vi "Image.vi"(2 "XRef":refnum<vi>, 3 "State In":T1={"Input Type"=variant(dbl 0.0), "Selection"=0, "Element Names"=[], "Type Strings"=[], "Element Types"=[]}) -> (0 "Image":picture)   [LabVIEW 2015, in "Construct-Tagged-Union.xnode"]
doc: "This ability VI is used to describe your XNode's appearance. The origin of Image corresponds to the top-left corner of your XNode. The bounds of your XNode are used to crop this image. If you want LabVIEW to update your image, you need to inform it through the UpdateImage or UpdateImageAndBounds replies. Any areas where you do not draw are transparent, so regions intended to appear white should be explicitly drawn.\n \n Remember to localize any strings that are part of your image.\n\nDefault behavior: None.\n\nThis ability does not provide UI and OS messages are not handled."
uses:
  Construct-Tagged-Union.xnode
  State.ctl
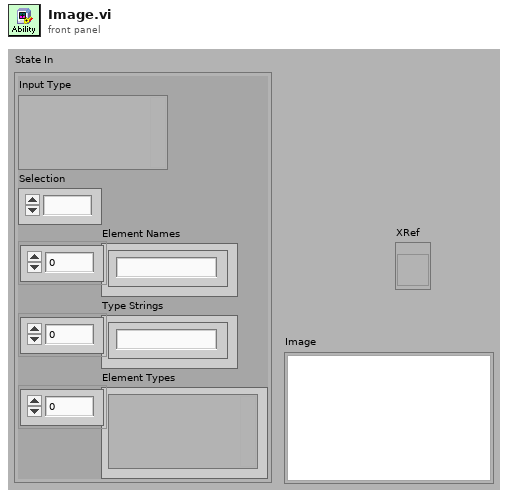
[diagram p1: front panel]
types:
  T1 = typedef "Construct-Tagged-Union.xnode/State.ctl" = cluster{"Input Type":variant, "Selection":i32, "Element Names":string[], "Type Strings":string[], "Element Types":variant[]}
  T2 = typedef "imagedata.ctl" = cluster{"image type":i32, "image depth":i32, "image":u8[], "mask":u8[], "colors":u32[], "Rectangle":cluster{"left":i16, "top":i16, "right":i16, "bottom":i16}}
  T3 = cluster{"left":i16, "top":i16, "right":i16, "bottom":i16}
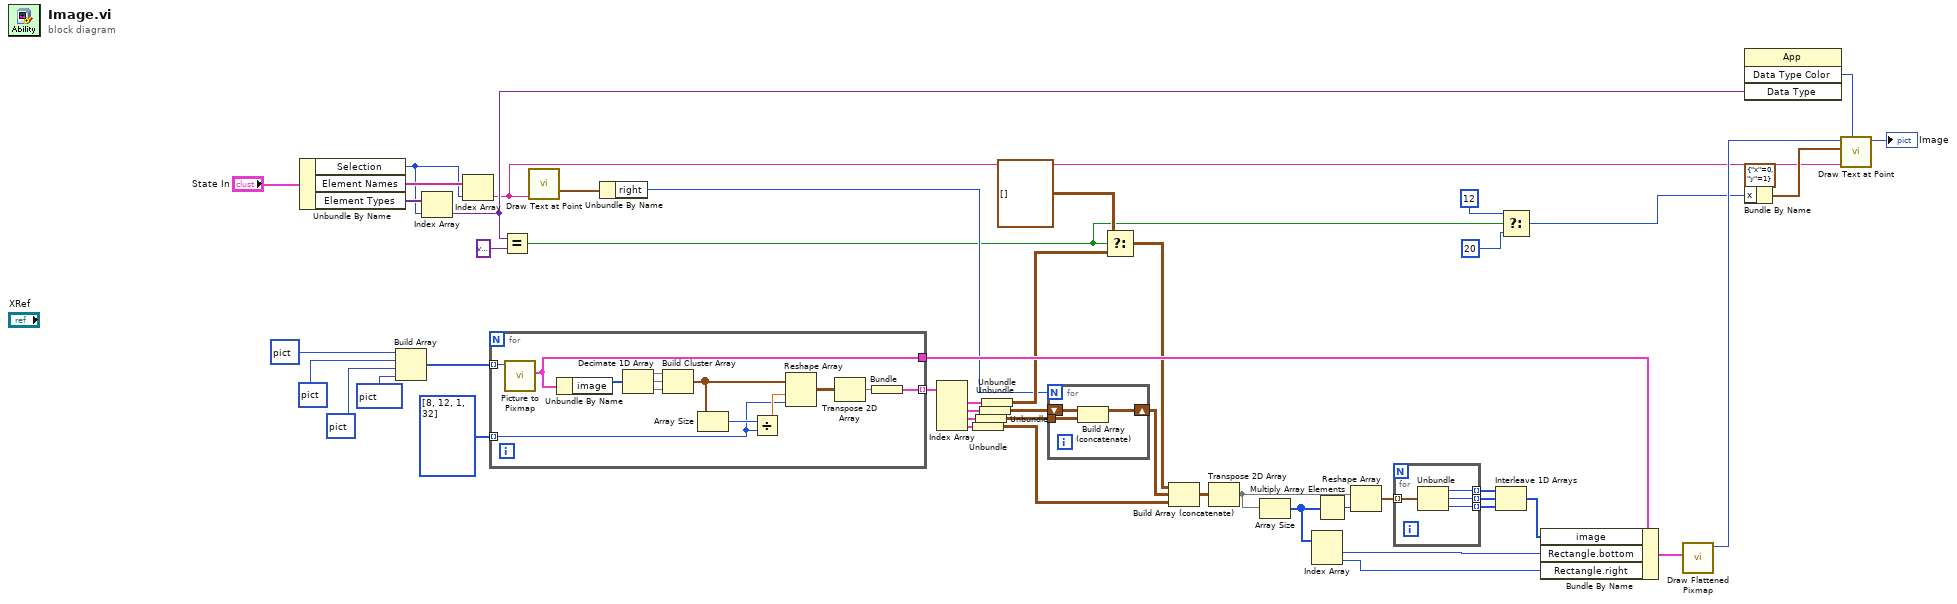
[diagram p0: block diagram]
diagram:
  n1 = Unbundle By Name("State In") -> ("Selection"=w42:i32, "Element Names"=w43:string[], "Element Types"=w44:variant[])
  n2 = Build Array(picture bytes[524] ("new picture"), picture bytes[714] ("new picture"), picture bytes[87] ("new picture"), picture bytes[1930] ("new picture")) -> (w20:picture[])
  n3 = Index Array(array=w44, index=w42) -> (element=w18:variant)
  n4 = Index Array(array=w43, index=w42) -> (element=w11:string)
  n5 = for {
    tunnel: w20 -> [w62] mode=indexing
    tunnel: i32[] [8, 12, 1, 32] -> [w54] mode=indexing
    tunnel: [w50] -> w40 mode=indexing
    tunnel: [w52] -> w25
    n6 = call <vilib>:"Picture to Pixmap.vi"("picture"=w62) -> ("image data"=w52:T2)  [unwired: 9 in, 1 out]
    n7 = Unbundle By Name(w52) -> ("image"=w58:u8[])
    n8 = Decimate 1D Array(w58) -> (w57:u8[], w55:u8[], w56:u8[])
    n9 = Build Cluster Array(w57, w55, w56) -> (w59:cluster{u8, u8, u8}[])
    n10 = Array Size(array=w59) -> (size(s)=w60:i32)
    n11 = Divide(x=w60, y=w54) -> (x/y=w61:dbl)
    n12 = Reshape Array(w59, w61, w54) -> (w53:cluster{u8, u8, u8}[][])
    n13 = Transpose 2D Array(2D array=w53) -> (transposed array=w51:cluster{u8, u8, u8}[][])
    n14 = Bundle(w51) -> (w50:cluster{cluster{u8, u8, u8}[][]})  [unwired: 1 in]
  }
  n15 = Equal?(x=w18, y=variant) -> (x = y?=w8:bool)
  n16 = call <vilib>:"Draw Text at Point.vi"("text"=w11) -> ("text rect"=w10:T3)  [unwired: 9 in, 1 out]
  n17 = Unbundle By Name(w10) -> ("right"=w9:i16)
  n18 = Index Array(array=w40) -> (element #1=w15:cluster{cluster{u8, u8, u8}[][]}, element #2=w38:cluster{cluster{u8, u8, u8}[][]}, element #3=w39:cluster{cluster{u8, u8, u8}[][]}, element #4=w36:cluster{cluster{u8, u8, u8}[][]})  [unwired: 4 in]
  n19 = Unbundle(w36) -> (w21:cluster{u8, u8, u8}[][])
  n20 = Unbundle(w39) -> (w22:cluster{u8, u8, u8}[][])
  n21 = Unbundle(w38) -> (w23:cluster{u8, u8, u8}[][])
  n22 = Unbundle(w15) -> (w14:cluster{u8, u8, u8}[][])
  n23 = for {
    N: w9 -> [_]
    shift-right: [w63] -> w37
    shift-left: w23 -> [w64]
    tunnel: w22 -> [w65]
    n24 = Build Array (concatenate)(w64, w65) -> (w63:cluster{u8, u8, u8}[][])
  }
  n25 = Select(t=cluster{u8, u8, u8}[][] [], s=w8, f=w14) -> (s? t:f=w13:cluster{u8, u8, u8}[][])
  n26 = Build Array (concatenate)(w13, w37, w21) -> (w35:cluster{u8, u8, u8}[][])
  n27 = Transpose 2D Array(2D array=w35) -> (transposed array=w26:cluster{u8, u8, u8}[][])
  n28 = Array Size(array=w26) -> (size(s)=w34:i32[])
  n29 = Index Array(array=w34) -> (element #1=w27:i32, element #2=w24:i32)  [unwired: 2 in]
  n30 = Multiply Array Elements(1:w34) -> (0:w33:i32)
  n31 = Reshape Array(w26, w33) -> (w32:cluster{u8, u8, u8}[])
  n32 = for {
    tunnel: w32 -> [w69] mode=indexing
    tunnel: [w68] -> w31 mode=indexing
    tunnel: [w67] -> w30 mode=indexing
    tunnel: [w66] -> w29 mode=indexing
    n33 = Unbundle(w69) -> (w68:u8, w67:u8, w66:u8)
  }
  n34 = Interleave 1D Arrays(w31, w30, w29) -> (w28:u8[])
  n35 = Select(t=12, s=w8, f=20) -> (s? t:f=w5:i32)
  n36 = Bundle By Name(cluster=w25, "image"=w28, "Rectangle.bottom"=w27, "Rectangle.right"=w24) -> (w19:T2)
  n37 = call <vilib>:"Draw Flattened Pixmap.vi"("image data"=w19) -> ("new picture"=w48:picture)  [unwired: 1 in, 7 out]
  n38 = invoke class="App" method="Data Type Color"("Data Type"=w18) -> ("Data Type Color"=w45:u32)  [unwired: 3 in, 3 out]
  n39 = Bundle By Name(cluster=cluster{"x":i16, "y":i16} {"x"=0, "y"=1} ("origin"), "x"=w5) -> (w46:cluster{"x":i16, "y":i16})
  n40 = call <vilib>:"Draw Text at Point.vi"("text color(black)"=w45, "text"=w11, "origin"=w46, "picture"=w48) -> ("new picture"=→"Image":picture)  [unwired: 6 in, 1 out]
